vi "Transmit.vi"(8 "error in (no error)":errorcluster, 10 "Transfer Group in":refnum<class "Transfer Group.lvclass">, 11 "DSFPlugin in":refnum<class "DSFPlugin Transceiver.lvclass">) -> (0 "error out":errorcluster, 2 "Transfer Group out":refnum<class "Transfer Group.lvclass">, 3 "DSFPlugin out":refnum<class "DSFPlugin Transceiver.lvclass">)   [LabVIEW 2017, in "DSFPluginTest.lvlib" / "DSFPlugin Transceiver.lvclass"]
uses:
  DSFPlugin Transceiver.lvclass
  builds/Data Sharing Framework/Current/Data Sharing Framework Core/DSF Core.lvlibp/Engine/Classes/Transfer Group/Transfer Group.lvclass
  DSFPlugin Transceiver.lvclass/DSFPlugin Transceiver.ctl
  builds/Data Sharing Framework/Current/Data Sharing Framework Core/DSF Core.lvlibp/Engine/Classes/Transceiver/Transceiver.lvclass
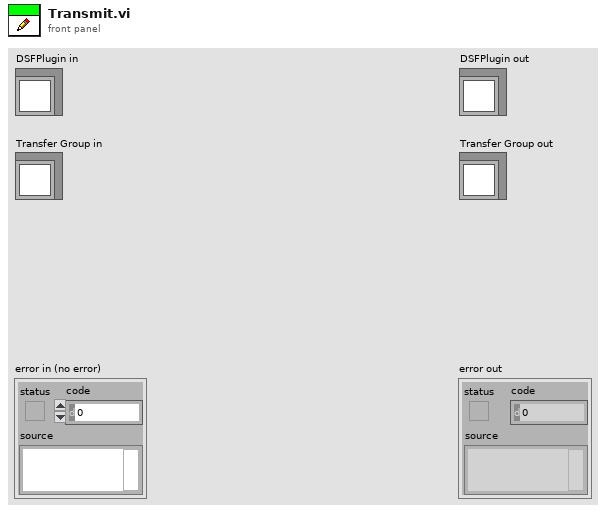
[diagram p1: front panel]
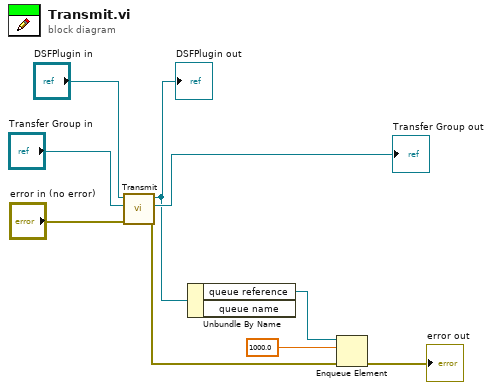
[diagram p0: block diagram]
diagram:
  n1 = call-parent "Transmit.vi"("error in (no error)"="error in (no error)", "Transfer Group in"="Transfer Group in", "Transceiver in"="DSFPlugin in") -> ("error out"=w2:errorcluster, "Transfer Group out"=→"Transfer Group out":refnum<class "Transfer Group.lvclass">, "Transceiver out"=w3:refnum<class "DSFPlugin Transceiver.lvclass">)  [unwired: 6 in]
  "DSFPlugin out" <- w3
  n2 = Unbundle By Name(w3) -> ("queue reference"=w6:refnum<queue>)  [unwired: 1 out]
  n3 = Enqueue Element(queue=w6, element=1000.0, error in (no error)=w2) -> (error out=→"error out":errorcluster)  [unwired: 1 in, 2 out]
